vi "data.vi"(8 "error in (no error)":errorcluster, 9 "AVG?":bool, 10 "Averaging Time":dbl, 11 "VISA resource name":refnum<visa-resource-name>) -> (0 "error out":errorcluster, 1 "SI":string, 2 "output":dbl, 3 "VISA resource name out":refnum<visa-resource-name>)   [LabVIEW 2009, in "Newport 1830-C.lvlib"]
doc: "AVG?=T, will return average of measurements taken 0.2 s apart for duration of averaging time.\nAVG?=F, will return one measurement."
uses:
  Newport 1830-C.lvlib
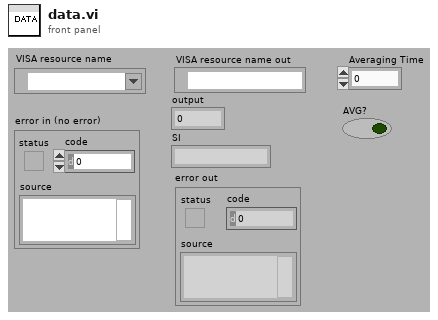
[diagram p1: front panel]
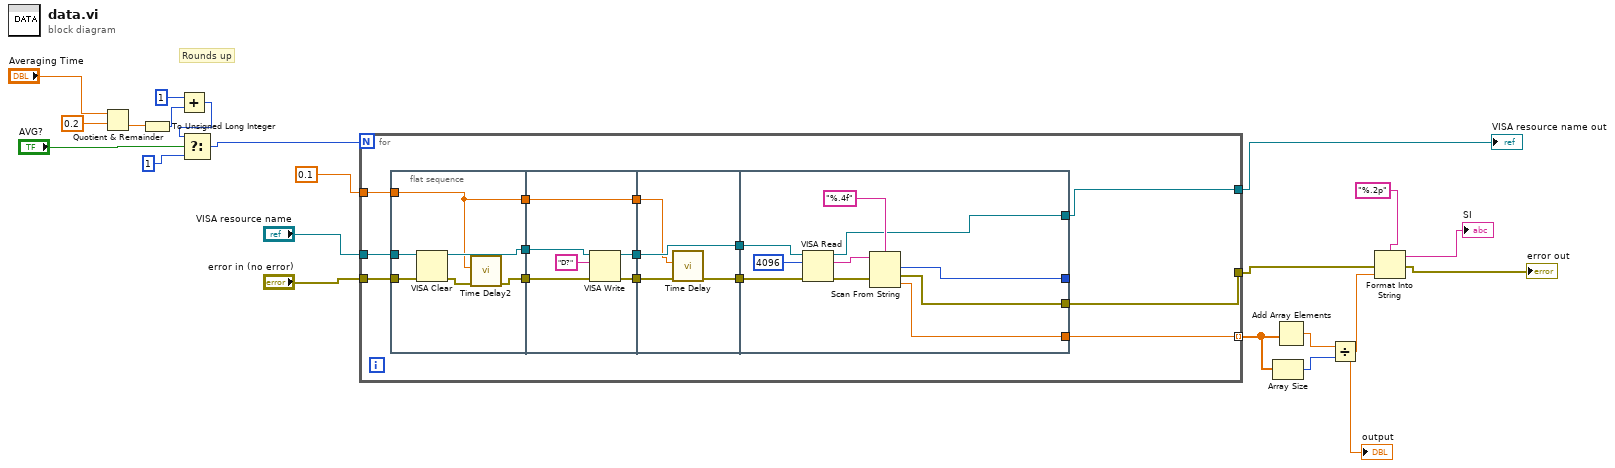
[diagram p0: block diagram]
diagram:
  # "Rounds up"
  n1 = Quotient & Remainder(x="Averaging Time", y=0.2) -> (floor(x/y)=w15:dbl)  [unwired: 1 out]
  n2 = To Unsigned Long Integer(number=w15) -> (unsigned 32bit integer=w3:u32)
  n3 = Add(x=u32 1, y=w3) -> (x+y=w1:u32)
  n4 = Select(t=w1, s="AVG?", f=u32 1 ("t")) -> (s? t:f=w14:u32)
  n5 = for {
    N: w14 -> [_]
    tunnel: "error in (no error)" -> [w27]
    tunnel: "VISA resource name" -> [w26]
    tunnel: 0.1 ("Delay Time (s)") -> [w25]
    tunnel: [w24] -> w11 mode=indexing
    tunnel: [w23] -> w7
    tunnel: [w22] -> w5
    n6 = flat-sequence {
      tunnel: [w37] -> w35
      tunnel: w27 -> [w41]
      tunnel: w26 -> [w40]
      tunnel: [w39] -> w34
      tunnel: w25 -> [w36]
      tunnel: [w36] -> w33
      tunnel: w35 -> [w46]
      tunnel: [w45] -> w32
      tunnel: [w44] -> w31
      tunnel: w34 -> [w43]
      tunnel: [w42] -> w30
      tunnel: w33 -> [w42]
      tunnel: w32 -> [w51]
      tunnel: [w50] -> w29
      tunnel: [w49] -> w28
      tunnel: w31 -> [w49]
      tunnel: w30 -> [w48]
      tunnel: w29 -> [w60]
      tunnel: w28 -> [w59]
      tunnel: [w54] -> w22
      tunnel: [w58] -> _
      tunnel: [w53] -> w24
      tunnel: [w52] -> w23
      frame #0 {
        n7 = VISA Clear(VISA resource name=w40, error in (no error)=w41) -> (VISA resource name out=w39:refnum<visa-resource-name>, error out=w38:errorcluster)
        n8 = call "Time Delay2"("error in (no error)"=w38, "Delay Time (s)"=w36) -> ("error out"=w37:errorcluster)  [unwired: 9 in]
      }
      frame #1 {
        n9 = VISA Write(VISA resource name=w43, write buffer="D?" ("command"), error in (no error)=w46) -> (VISA resource name out=w44:refnum<visa-resource-name>, error out=w45:errorcluster)  [unwired: 1 out]
      }
      frame #2 {
        n10 = call "Time Delay"("error in (no error)"=w51, "Delay Time (s)"=w48) -> ("error out"=w50:errorcluster)  [unwired: 9 in]
      }
      frame #3 {
        n11 = VISA Read(VISA resource name=w59, byte count=u32 4096, error in (no error)=w60) -> (VISA resource name out=w54:refnum<visa-resource-name>, read buffer=w56:string, error out=w55:errorcluster)  [unwired: 1 out]
        n12 = Scan From String(format string="%.4f", input string=w56, error in=w55) -> (offset past scan=w58:u32, error out=w52:errorcluster, output 1=w53:dbl)  [unwired: 2 in, 1 out]
      }
    }
  }
  "VISA resource name out" <- w5
  n13 = Array Size(array=w11) -> (size(s)=w10:i32)
  n14 = Add Array Elements(numeric array=w11) -> (sum=w9:dbl)
  n15 = Divide(x=w9, y=w10) -> (x/y=w8:dbl)
  "output" <- w8
  n16 = Format Into String(format string="%.2p", error in=w7, w8) -> (resulting string=→"SI":string, error out=→"error out":errorcluster)  [unwired: 1 in]
